vi "host.vi"() -> ()   [LabVIEW 2020]
uses:
  <vilib>/Analysis/baseanly.llb/Real Dot Product.vi
  <vilib>/Analysis/baseanly.llb/Real A x B.vi
  <vilib>/Analysis/Matrix/Numeric/Conversions/Matrix To Array - RM.vi
  <vilib>/FPGAPlugInAG/cRIO-9035/niLvFpga_Open_cRIO-9035.vi
  <vilib>/rvi/interface/common/dynamic/niFpgaDynamicAddResources.vi
  <vilib>/Utility/error.llb/Error Cluster From Error Code.vi
  <vilib>/rvi/errors/niLvFpgaAdjustHostInterfaceError.vi
  <vilib>/FPGAPlugInAG/Dynamic/niLvFpga_Run_Dynamic.vi
  <vilib>/FPGAPlugInAG/Dynamic/niLvFpga_Close_Dynamic.vi
  <vilib>/rvi/interface/nirviOpenFPGA/nirviOpenFPGA.xnode
  FPGA Bitfiles/v1.2_FPGATarget_target_O2QBpR2QsaI.lvbitx
  target.vi
  <vilib>/rvi/interface/nirviMethod/nirviMethod.xnode
  <vilib>/rvi/interface/nirviCloseFPGA/nirviCloseFPGA.xnode
  <vilib>/FPGAPlugInAG/Dynamic/niLvFpga_WriteFifo_Dynamic.vi
  <vilib>/rvi/errors/niLvFpgaMergeErrorWithErrorCode.vi
  <vilib>/Analysis/NI_AALBase.lvlib
  <vilib>/Analysis/Matrix/NI_Matrix.lvlib
  <vilib>/FPGAPlugInAG/Dynamic/niLvFpga_ReadFifo_Dynamic.vi
panel:
  out "X * Y":dbl format="%.6f"
  out "elements in B":i32
  out "elements in A":i32
  out "sum of error":dbl
  out "C - FPGA code":sgl[][](array[numeric])
  out "elements in C":i32
  out "C - Real":dbl[][](array[numeric])
  out "B":sgl[][](array[numeric])
  out "A":sgl[][](array[numeric])
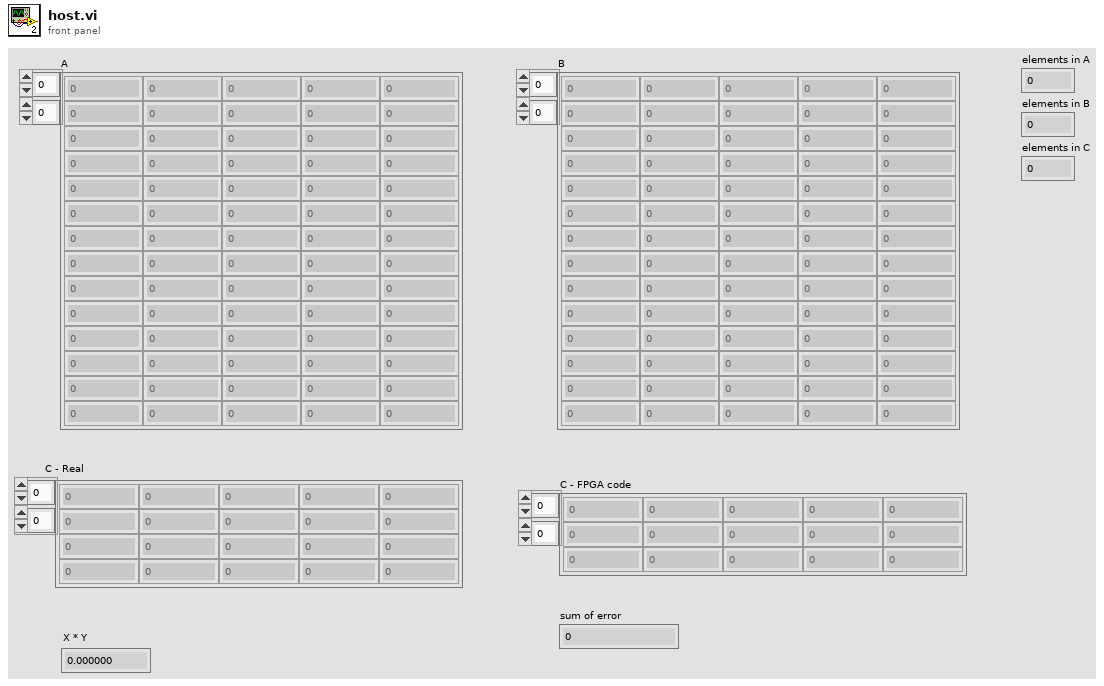
[diagram p1: front panel]
types:
  T1 = typedef "NI_Matrix.lvlib/RealMatrix.ctl" = dbl[][]
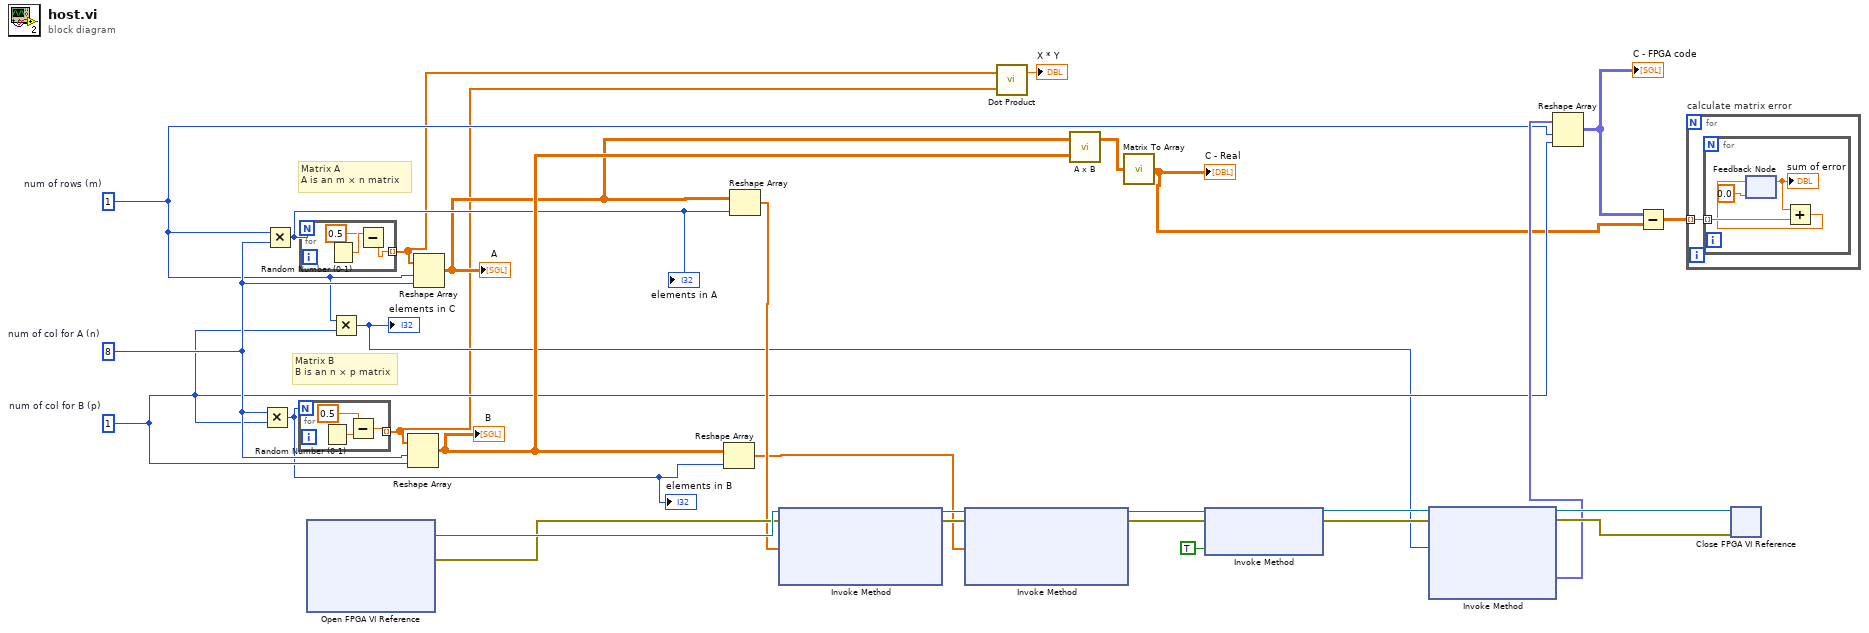
[diagram p0: block diagram]
diagram:
  w8 = 1  # num of col for B (p)
  w15 = 8  # num of col for A (n)
  w9 = 1  # num of rows (m)
  # "Matrix B\nB is an n × p matrix"
  # "Matrix A\nA is an m × n matrix"
  n1 = Multiply(x=w15, y=w8) -> (x*y=w5:i32)
  "elements in B" <- w5
  n2 = Multiply(x=w9, y=w15) -> (x*y=w16:i32)
  "elements in A" <- w16
  n3 = for {
    N: w5 -> [_]
    tunnel: [w31] -> w2 mode=indexing
    n4 = Random Number (0-1)() -> (number: 0 to 1=w32:dbl)
    n5 = Subtract(x=w32, y=sgl 0.5) -> (x-y=w31:sgl)
  }
  n6 = for {
    N: w16 -> [_]
    tunnel: [w34] -> w3 mode=indexing
    n7 = Random Number (0-1)() -> (number: 0 to 1=w35:dbl)
    n8 = Subtract(x=w35, y=sgl 0.5) -> (x-y=w34:sgl)
  }
  n9 = xnode "Open FPGA VI Reference"() -> ("FPGA VI Reference Out"=w28:refnum<k20>, "error out"=w27:errorcluster)  [unwired: 2 in]
  n10 = Multiply(x=w9, y=w8) -> (x*y=w6:i32)
  "elements in C" <- w6
  n11 = Reshape Array(w2, w15, w8) -> (w18:sgl[][])
  "B" <- w18
  n12 = Reshape Array(w3, w9, w15) -> (w4:sgl[][])
  "A" <- w4
  n13 = Reshape Array(w18, w5) -> (w13:sgl[])
  n14 = Reshape Array(w4, w16) -> (w14:sgl[])
  n15 = xnode "Invoke Method"("FPGA VI Reference In"=w28, "error in"=w27, "Data"=w14) -> ("FPGA VI Reference Out"=w22:refnum<k20>, "error out"=w21:errorcluster)  [unwired: 1 in, 1 out]
  n16 = xnode "Invoke Method"("FPGA VI Reference In"=w22, "error in"=w21, "Data"=w13) -> ("FPGA VI Reference Out"=w20:refnum<k20>, "error out"=w19:errorcluster)  [unwired: 1 in, 1 out]
  n17 = call-poly <vilib>:"Dot Product.vi"("Y Vector"=w2, "X Vector"=w3) -> ("X * Y"=→"X * Y":dbl)  [unwired: 1 out]
  n18 = call-poly <vilib>:"A x B.vi"("B"=w18, "A"=w4) -> ("A x B"=w17:T1)  [unwired: 1 out]
  n19 = call-poly <vilib>:"Matrix To Array.vi"("Real Matrix"=w17) -> ("Real 2D Array"=w7:dbl[][])
  "C - Real" <- w7
  n20 = xnode "Invoke Method"("FPGA VI Reference In"=w20, "error in"=w19, "Wait Until Done (F)"=TRUE) -> ("FPGA VI Reference Out"=w26:refnum<k20>, "error out"=w25:errorcluster)
  n21 = xnode "Invoke Method"("FPGA VI Reference In"=w26, "error in"=w25, "Number of Elements"=w6) -> ("FPGA VI Reference Out"=w24:refnum<k20>, "error out"=w23:errorcluster, "Data"=w10:fxp<+/-,20,10>[])  [unwired: 1 in, 1 out]
  n22 = Reshape Array(w10, w9, w8) -> (w12:fxp<+/-,20,10>[][])
  "C - FPGA code" <- w12
  n23 = Subtract(x=w12, y=w7) -> (x-y=w11:dbl[][])
  n24 = for "calculate matrix error" {
    tunnel: w11 -> [w36] mode=indexing
    n25 = for {
      tunnel: w36 -> [w40] mode=indexing
      n26 = feedback #1(0.0) -> (w38:dbl)
      "sum of error" <- w38
      n27 = Add(x=w38, y=w40) -> (x+y=w39:dbl)
      n28 = feedback-in #1(w39) -> ()
    }
  }
  n29 = xnode "Close FPGA VI Reference"("FPGA VI Reference In"=w24, "error in"=w23) -> ()  [unwired: 1 out]
